vi "2D Cubic Path.vi"(0 "Pose i":cluster{"X":dbl, "Y":dbl, "Theta[deg]":dbl}, 1 "Pose f":cluster{"X":dbl, "Y":dbl, "Theta[deg]":dbl}, 2 "Constraints":cluster{"Vmax":dbl, "Amax":dbl}={"Vmax"=100.0, "Amax"=200.0}, 3 "Number Of Points":i32=100, 4 "K":dbl(slide) scale=-500.0..500.0) -> (5 "Total Time":dbl, 6 "Motion Profile":T1(array[cluster]))   [LabVIEW 2016]
uses:
  <vilib>/Analysis/polynomials.llb/Scalar Polynomial Evaluation (DBL).vi
  <vilib>/Analysis/NI_AALPro.lvlib
panel:
  in  "b":dbl=25.0 format="%#_13g"
  out "Points":T2(array[cluster])
  out "Length":dbl
  out "Spline Y":dbl[](array[numeric])
  out "Spline X":dbl[](array[numeric])
  out "XY Graph":cluster{"X":dbl, "Y":dbl}[](graph)
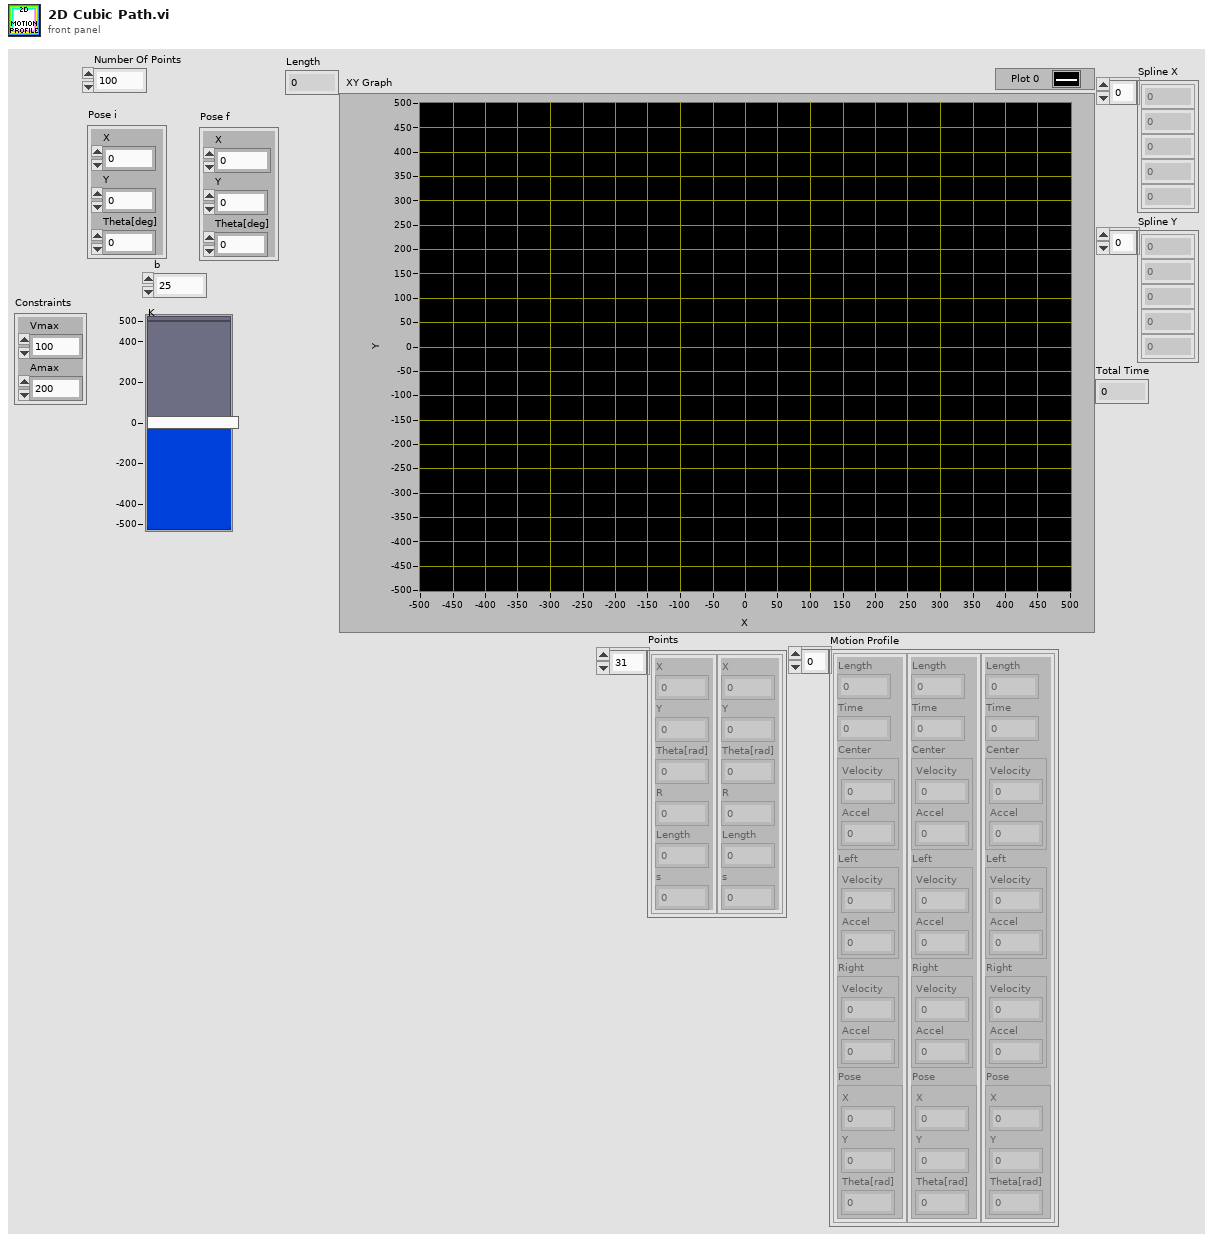
[diagram p1: front panel]
types:
  T1 = cluster{"Length":dbl, "Time":dbl, "Center":cluster{"Velocity":dbl, "Accel":dbl}, "Left":cluster{"Velocity":dbl, "Accel":dbl}, "Right":cluster{"Velocity":dbl, "Accel":dbl}, "Pose":cluster{"X":dbl, "Y":dbl, "Theta[rad]":dbl}}[]
  T2 = cluster{"X":dbl, "Y":dbl, "Theta[rad]":dbl, "R":dbl, "Length":dbl, "s":dbl}[]
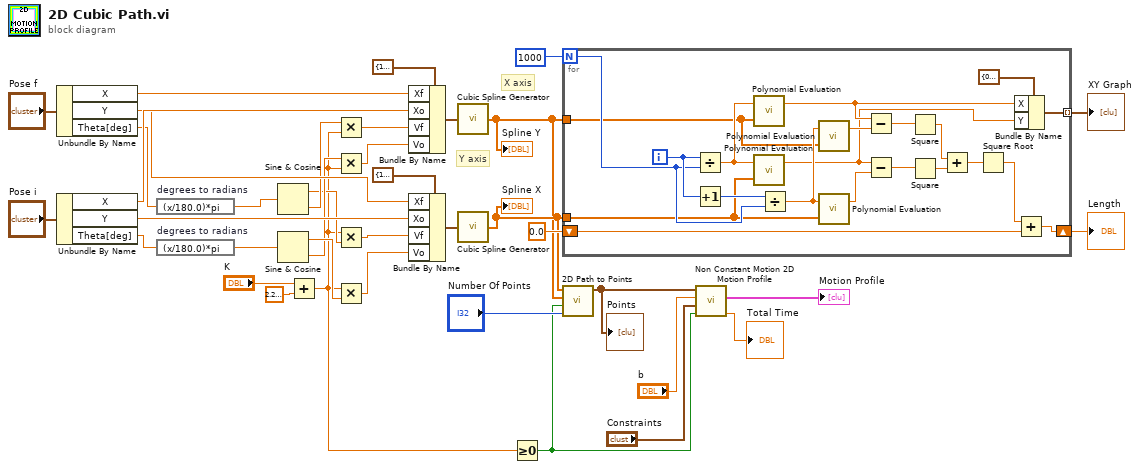
[diagram p0: block diagram]
diagram:
  # "Y axis"
  # "X axis"
  n1 = Unbundle By Name("Pose f") -> ("X"=w32:dbl, "Y"=w28:dbl, "Theta[deg]"=w19:dbl)
  n2 = Unbundle By Name("Pose i") -> ("X"=w31:dbl, "Y"=w27:dbl, "Theta[deg]"=w36:dbl)
  n3 = expression code="(x/180.0)*pi" "degrees to radians"(w19) -> (w20:dbl)
  n4 = expression code="(x/180.0)*pi" "degrees to radians"(w36) -> (w35:dbl)
  n5 = Sine & Cosine(0:w20) -> (1:w21:dbl, 2:w22:dbl)
  n6 = Sine & Cosine(0:w35) -> (1:w26:dbl, 2:w25:dbl)
  n7 = Add(x="K", y=2.220446049250313e-16) -> (x+y=w3:dbl)
  n8 = Multiply(x=w22, y=w3) -> (x*y=w17:dbl)
  n9 = Multiply(x=w25, y=w3) -> (x*y=w23:dbl)
  n10 = Multiply(x=w3, y=w21) -> (x*y=w18:dbl)
  n11 = Multiply(x=w3, y=w26) -> (x*y=w24:dbl)
  n12 = Bundle By Name(cluster=cluster{"Xf":dbl, "Xo":dbl, "Vf":dbl, "Vo":dbl} {"Xf"=100.0, "Xo"=0.0, "Vf"=0.0, "Vo"=0.0} ("Configurations"), "Xf"=w32, "Xo"=w31, "Vf"=w17, "Vo"=w23) -> (w34:cluster{"Xf":dbl, "Xo":dbl, "Vf":dbl, "Vo":dbl})
  n13 = Bundle By Name(cluster=cluster{"Xf":dbl, "Xo":dbl, "Vf":dbl, "Vo":dbl} {"Xf"=100.0, "Xo"=0.0, "Vf"=0.0, "Vo"=0.0} ("Configurations"), "Xf"=w28, "Xo"=w27, "Vf"=w18, "Vo"=w24) -> (w29:cluster{"Xf":dbl, "Xo":dbl, "Vf":dbl, "Vo":dbl})
  n14 = call "Cubic Spline Generator.vi"("Configurations"=w34) -> ("Spline"=w12:dbl[])
  "Spline Y" <- w12
  n15 = call "Cubic Spline Generator.vi"("Configurations"=w29) -> ("Spline"=w13:dbl[])
  "Spline X" <- w13
  n16 = Greater Or Equal To 0?(x=w3) -> (x >= 0?=w4:bool)
  n17 = for {
    N: 1000 -> [w53]
    tunnel: w12 -> [w52]
    tunnel: w13 -> [w51]
    tunnel: [w57] -> w10 mode=indexing
    shift-right: [w40] -> w14
    shift-left: 0.0 -> [w39]
    i -> [w55]
    n18 = Divide(x=w55, y=w53) -> (x/y=w59:dbl)
    n19 = Increment(x=w55) -> (x+1=w54:i32)
    n20 = call-poly <vilib>:"Polynomial Evaluation.vi"("P(x)"=w52, "a"=w59) -> ("P(a)"=w50:dbl)  [unwired: 1 out]
    n21 = call-poly <vilib>:"Polynomial Evaluation.vi"("P(x)"=w51, "a"=w59) -> ("P(a)"=w48:dbl)  [unwired: 1 out]
    n22 = Divide(x=w54, y=w53) -> (x/y=w56:dbl)
    n23 = call-poly <vilib>:"Polynomial Evaluation.vi"("P(x)"=w52, "a"=w56) -> ("P(a)"=w49:dbl)  [unwired: 1 out]
    n24 = call-poly <vilib>:"Polynomial Evaluation.vi"("P(x)"=w51, "a"=w56) -> ("P(a)"=w47:dbl)  [unwired: 1 out]
    n25 = Subtract(x=w50, y=w49) -> (x-y=w45:dbl)
    n26 = Subtract(x=w48, y=w47) -> (x-y=w46:dbl)
    n27 = Square(x=w45) -> (x^2=w44:dbl)
    n28 = Square(x=w46) -> (x^2=w43:dbl)
    n29 = Add(x=w44, y=w43) -> (x+y=w42:dbl)
    n30 = Square Root(x=w42) -> (sqrt(x)=w41:dbl)
    n31 = Bundle By Name(cluster=cluster{"X":dbl, "Y":dbl} {"X"=0.0, "Y"=0.0} ("XY Graph 2"), "X"=w50, "Y"=w48) -> (w57:cluster{"X":dbl, "Y":dbl})
    n32 = Add(x=w41, y=w39) -> (x+y=w40:dbl)
  }
  "XY Graph" <- w10
  "Length" <- w14
  n33 = call "2D Path to Points.vi"("Number Of Points"="Number Of Points", "Forward"=w4, "Spline Y"=w12, "Spline X"=w13) -> ("Points"=w9:T2)  [unwired: 7 in]
  "Points" <- w9
  n34 = call "Non Constant Motion 2D Motion Profile.vi"("Forward?"=w4, "Wheel Constraints"="Constraints", "b"="b", "Points"=w9) -> ("Total Time"=→"Total Time":dbl, "Moition Profiel"=→"Motion Profile":T1)  [unwired: 6 in]
